vi "programa 1 DAQ.vi"() -> ()   [LabVIEW 2011]
panel:
  in  "on/off":bool
  in  "llenar":i32(knob) scale=0.0..5.0
  out "tanque":i32(slide) scale=0.0..10.0
  out "foco":bool
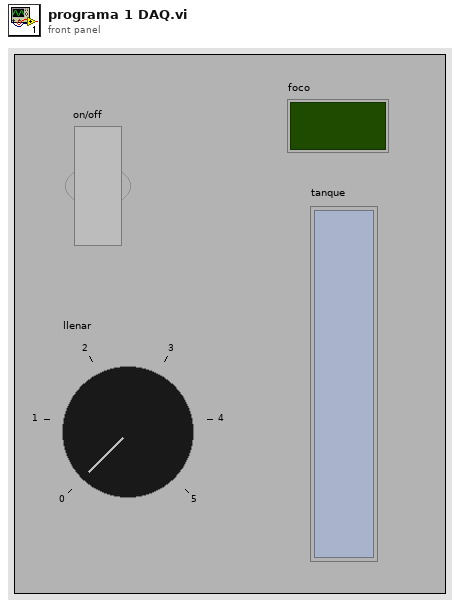
[diagram p1: front panel]
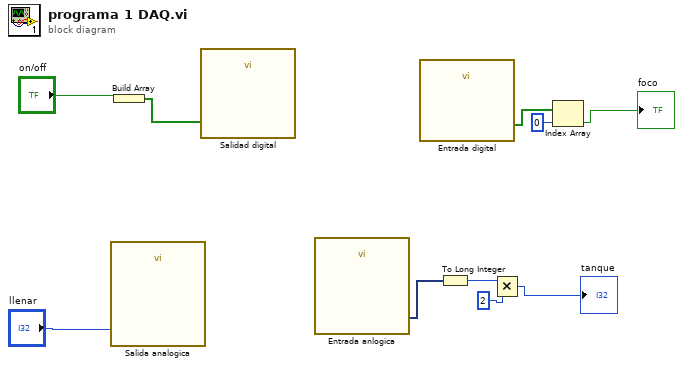
[diagram p0: block diagram]
diagram:
  n1 = call "Salida analogica"("data"="llenar") -> ()  [unwired: 17 in, 2 out]
  n2 = Build Array("on/off") -> (w4:bool[])
  n3 = call "Salidad digital"("data"=w4) -> ()  [unwired: 17 in, 2 out]
  n4 = call "Entrada anlogica"() -> ("data"=w7:dynamicdata)  [unwired: 17 in, 2 out]
  n5 = call "Entrada digital"() -> ("data"=w3:bool[])  [unwired: 17 in, 2 out]
  n6 = To Long Integer(number=w7) -> (32bit integer=w8:i32)
  n7 = Multiply(x=w8, y=2) -> (x*y=→"tanque":i32)
  n8 = Index Array(array=w3, index=0) -> (element=→"foco":bool)
